vi "create.ModifyOrderBase.vi"(8 "error in (no error)":errorcluster, 11 "ModifyOrderBase in":refnum<class "ModifyOrderBase.lvclass">) -> (0 "error out":errorcluster, 3 "ModifyOrderBase out":refnum<class "ModifyOrderBase.lvclass">)   [LabVIEW 2020, in "ModifyOrderBase.lvclass"]
uses:
  ModifyOrderBase.lvclass
  FieldSpec.ctl
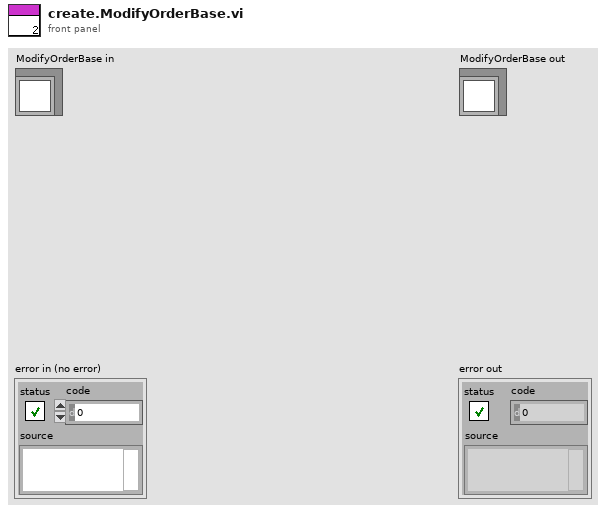
[diagram p1: front panel]
types:
  T1 = typedef "FieldSpec.ctl" = cluster{"Name":string, "Offset":i32, "Length":i32, "FieldType":enum16{"Alphanumeric", "Binary", "BinaryLongPrice", "BinaryShortPrice", "BitField", "PrintableAscii", "Value"}, "FieldValue":variant}
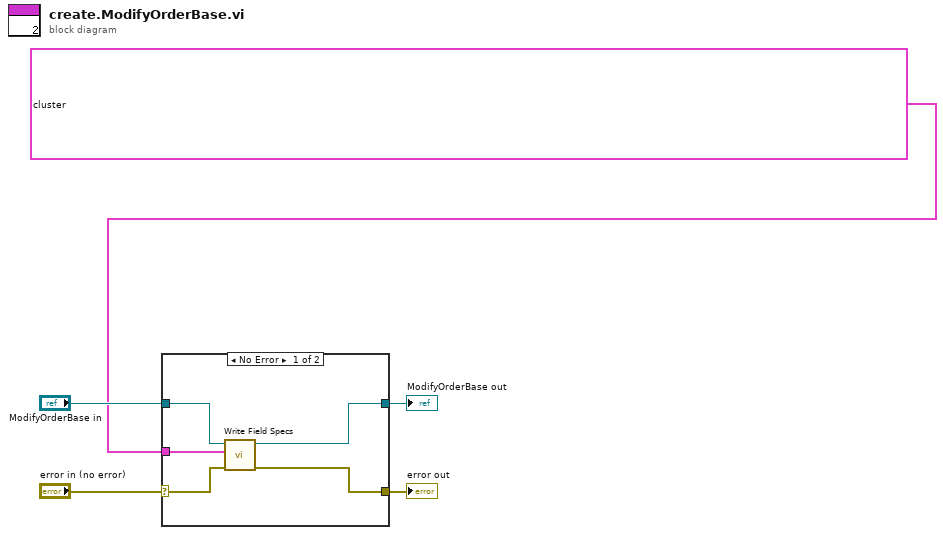
[diagram p0: block diagram]
diagram:
  n1 = case shown="No Error" "error in (no error)" {
    selector: "error in (no error)" -> [w8 w12]
    tunnel: [w9 w12] -> w4
    tunnel: [w7 w11] -> w2
    tunnel: "ModifyOrderBase in" -> [w10 w11]
    tunnel: T1[] [{"Name"="Length", "Offset"=0, "Length"=1, "FieldType"=enum."Binary", "FieldValue"=variant}, {"Name"="MessageType", "Offset"=1, "Length"=1, "FieldType"=enum."Value", "FieldValue"=variant}, {"Name"="Time Offset", "Offset"=2, "Length"=4, "FieldType"=enum."Binary", "FieldValue"=variant}, {"Name"="Order Id", "Offset"=6, "Length"=8, "FieldType"=enum."Binary", "FieldValue"=variant}, {"Name"="Quantity", "Offset"=14, "Length"=4, "FieldType"=enum."Binary", "FieldValue"=variant}, {"Name"="Price", "Offset"=18, "Length"=8, "FieldType"=enum."BinaryLongPrice", "FieldValue"=variant}, {"Name"="Modify Flags", "Offset"=26, "Length"=1, "FieldType"=enum."BitField", "FieldValue"=variant}] ("appended array") -> [w6 _]
    frame No Error {
      n2 = call-dynamic "Write Field Specs.vi"("error in (no error)"=w8, "Field Specs"=w6, "MessageBase in"=w10) -> ("error out"=w9:errorcluster, "MessageBase out"=w7:refnum<class "ModifyOrderBase.lvclass">)  [unwired: 7 in]
    }
    frame Error {
    }
  }
  "error out" <- w4
  "ModifyOrderBase out" <- w2
